vi "数据导出Excel.vi"(8 "error in (no error)":errorcluster caption="错误输入（无错误）", 10 "text data":string[][](array[string]) caption="文本数据", 11 "default name":string="历史数据.xlsx" caption="默认名称") -> (0 "error out":errorcluster caption="错误输出", 3 "布尔":bool)   [LabVIEW 2016, in "数据查询.lvlib"]
uses:
  <vilib>/Utility/sysdir.llb/System Directory Type.ctl
  <vilib>/Utility/NIReport.llb/Append Text Table to Report (wrap).vi
  <vilib>/Utility/NIReport.llb/NI_report.lvclass
  <vilib>/Utility/NIReport.llb/Excel/NI_Excel.lvclass
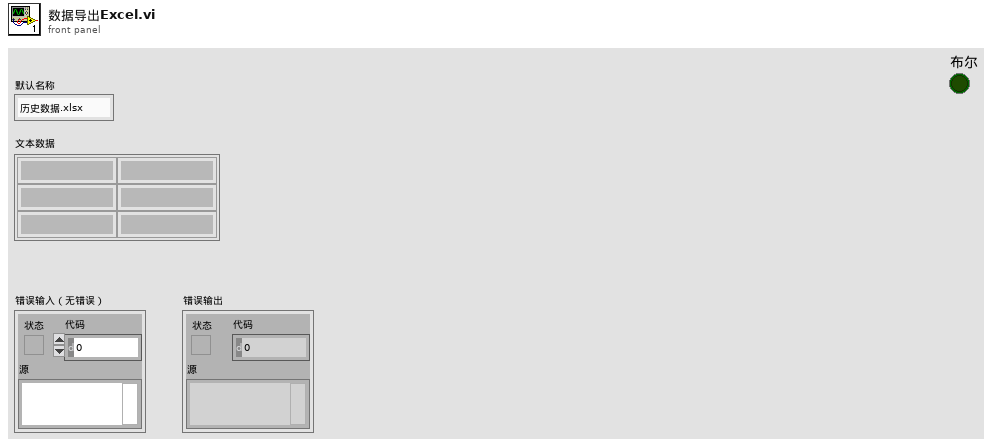
[diagram p1: front panel]
types:
  T1 = typedef "System Directory Type.ctl" = i32
  T2 = enum16{"maximized", "minimized", "normal", "no change"}
  T3 = enum16{"Standard Report", "HTML", "Word", "Excel"}
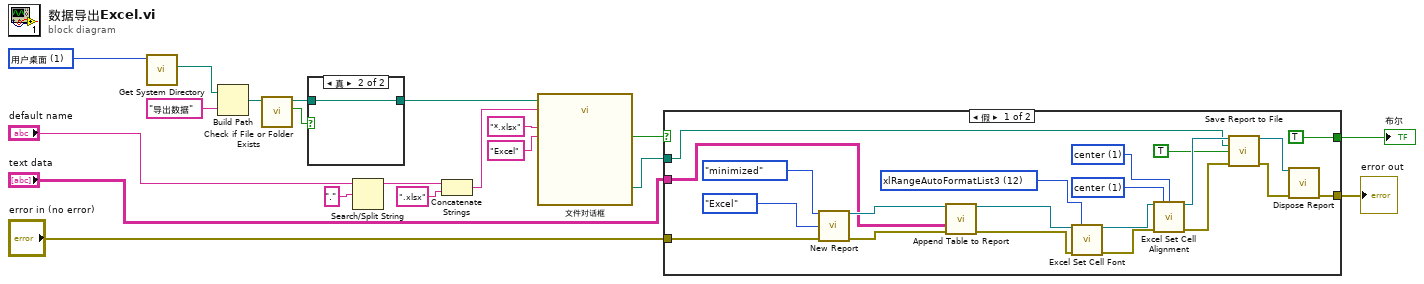
[diagram p0: block diagram]
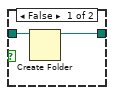
[diagram p2: hidden frame]
diagram:
  w7 = T1 1 items=["用户目录"=0, "用户桌面"=1, "用户文档"=2, "用户应用程序数据"=3, "用户设置"=4, "用户临时目录"=5, "公共文档"=6, "公共应用程序数据"=7, "公共设置"=8, "公共缓存"=13, "系统核心库"=9, "系统安装库"=10, "应用程序文件"=11, "启动盘根目录"=12] ("system directory type")
  n1 = call <vilib>:"Get System Directory.vi"("system directory type"=w7) -> ("system directory"=w6:path)  [unwired: 10 in]
  n2 = Build Path(base path=w6, name or relative path="导出数据" ("名称或相对路径")) -> (appended path=w4:path)
  n3 = call <vilib>:"Check if File or Folder Exists.vi"("path"=w4) -> ("file or folder exists?"=w3:bool, "dup path"=w2:path)  [unwired: 8 in, 1 out]
  n4 = case shown="真" w3 {
    tunnel: w2 -> [w22 w23]
    tunnel: [w21 w23] -> w1
    frame False {
      n5 = Create Folder(path (use dialog)=w22) -> (created path=w21:path)  [unwired: 2 in, 2 out]
    }
    frame True {
    }
  }
  n6 = Search/Split String(string="default name", search string/char (-)="." ("搜索字符串/字符(-)")) -> (substring before match=w10:string)  [unwired: 1 in, 2 out]
  n7 = Concatenate Strings(w10, ".xlsx" ("pattern (all files)")) -> (w8:string)
  n8 = call "文件对话框"("start path"=w1, "default name"=w8, "pattern (all files)"="*.xlsx", "pattern label"="Excel") -> ("selected path"=w17:path, "cancelled"=w18:bool)  [unwired: 8 in, 2 out]
  n9 = case shown="假" w18 {
    tunnel: w17 -> [w29 _]
    tunnel: "error in (no error)" -> [w28 w45]
    tunnel: [w27 w45] -> w15
    tunnel: "text data" -> [w25 _]
    tunnel: [TRUE _] -> w13
    frame False {
      w30 = 1 items=["left", "center", "right"] ("horizontal alignment (left)")
      w31 = 1 items=["top", "center", "bottom"] ("vertical alignment (top)")
      w34 = 12 items=["xlRangeAutoFormat3DEffects1"=13, "xlRangeAutoFormat3DEffects2"=14, "xlRangeAutoFormatAccounting1"=4, "xlRangeAutoFormatAccounting2"=5, "xlRangeAutoFormatAccounting3"=6, "xlRangeAutoFormatAccounting4"=17, "xlRangeAutoFormatClassic1"=1, "xlRangeAutoFormatClassic2"=2, "xlRangeAutoFormatClassic3"=3, "xlRangeAutoFormatColor1"=7, "xlRangeAutoFormatColor2"=8, "xlRangeAutoFormatColor3"=9, "xlRangeAutoFormatList1"=10, "xlRangeAutoFormatList2"=11, "xlRangeAutoFormatList3"=12, "xlRangeAutoFormatLocalFormat1"=15, "xlRangeAutoFormatLocalFormat2"=16, "xlRangeAutoFormatLocalFormat3"=19, "xlRangeAutoFormatLocalFormat4"=20, "xlRangeAutoFormatReport1"=21, "xlRangeAutoFormatReport2"=22, "xlRangeAutoFormatReport3"=23, "xlRangeAutoFormatReport4"=24, "xlRangeAutoFormatReport5"=25, "xlRangeAutoFormatReport6"=26, "xlRangeAutoFormatReport7"=27, "xlRangeAutoFormatReport8"=28, "xlRangeAutoFormatReport9"=29, "xlRangeAutoFormatReport10"=30, "xlRangeAutoFormatClassicPivotTable"=31, "xlRangeAutoFormatTable1"=32, "xlRangeAutoFormatTable2"=33, "xlRangeAutoFormatTable3"=34, "xlRangeAutoFormatTable4"=35, "xlRangeAutoFormatTable5"=36, "xlRangeAutoFormatTable6"=37, "xlRangeAutoFormatTable7"=38, "xlRangeAutoFormatTable8"=39, "xlRangeAutoFormatTable9"=40, "xlRangeAutoFormatTable10"=41, "xlRangeAutoFormatPTNone"=42, "xlRangeAutoFormatNone"=-4142, "xlRangeAutoFormatSimple"=-4154] ("auto format")
      n10 = call <vilib>:"New Report.vi"("window state (normal)"=T2."minimized", "report type"=T3."Excel", "error in (no error)"=w28) -> ("report out"=w40:refnum<class "NI_report.lvclass">, "error out"=w39:errorcluster)  [unwired: 11 in]
      n11 = call-poly <vilib>:"Append Table to Report.vi"("report in"=w40, "text data"=w25, "error in (no error)"=w39) -> ("report out"=w38:refnum<class "NI_report.lvclass">, "error out"=w37:errorcluster)  [unwired: 9 in, 2 out]
      n12 = call <vilib>:"Excel Set Cell Font.vi"("report in"=w38, "auto format"=w34, "error in (no error)"=w37) -> ("report out"=w33:refnum<class "NI_report.lvclass">, "error out"=w32:errorcluster)  [unwired: 11 in]
      n13 = call <vilib>:"Excel Set Cell Alignment.vi"("report in"=w33, "vertical alignment (top)"=w31, "horizontal alignment (left)"=w30, "error in (no error)"=w32) -> ("report out"=w36:refnum<class "NI_report.lvclass">, "error out"=w35:errorcluster)  [unwired: 10 in]
      n14 = call-dynamic "Save Report to File.vi"("report in"=w36, "report file path"=w29, "prompt to replace? (F)"=TRUE, "error in (no error)"=w35) -> ("report out"=w42:refnum<class "NI_report.lvclass">, "error out"=w41:errorcluster)  [unwired: 10 in]
      n15 = call-dynamic "Dispose Report.vi"("report in"=w42, "error in (no error)"=w41) -> ("error out"=w27:errorcluster)  [unwired: 13 in]
    }
    frame True {
    }
  }
  "error out" <- w15
  "布尔" <- w13
